vi "OutSineAmpSet.vi"(0 "SR865 in":T1, 2 "Amplitude":dbl caption="Amplitude, V", 5 "error in":errorcluster) -> (14 "SR865 out":T1, 19 "error out":errorcluster)   [LabVIEW 2018]
uses:
  SR865.ctl
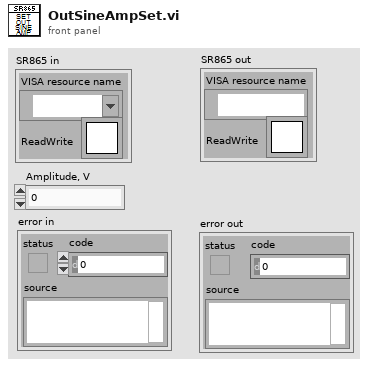
[diagram p1: front panel]
types:
  T1 = typedef "SR865.ctl" = cluster{"VISA resource name":refnum<visa-resource-name>, "ReadWrite":T2}
  T2 = typedef "Semaphore RefNum" = refnum<k1>
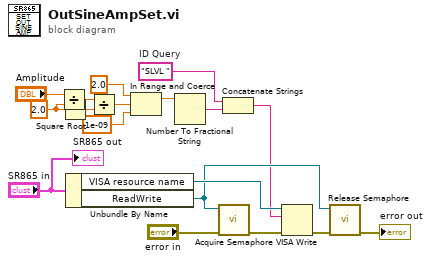
[diagram p0: block diagram]
diagram:
  w3 = 2.0 ("y")
  w9 = "SLVL "  # ID Query
  n1 = Divide(x="Amplitude", y=w3) -> (x/y=w5:dbl)
  n2 = Square Root(x=w3) -> (sqrt(x)=w4:dbl)
  n3 = Unbundle By Name("SR865 in") -> ("VISA resource name"=w17:refnum<visa-resource-name>, "ReadWrite"=w13:T2)
  n4 = Divide(x=w5, y=w4) -> (x/y=w2:dbl)
  n5 = In Range and Coerce(upper limit=2.0, x=w2, lower limit=1e-09) -> (coerced(x)=w10:dbl)  [unwired: 1 out]
  n6 = Number To Fractional String(number=w10) -> (F-format string=w8:string)  [unwired: 3 in]
  n7 = call <vilib>:"Acquire Semaphore.vi"("error in (no error)"="error in", "semaphore"=w13) -> ("error out"=w16:errorcluster)  [unwired: 3 in, 2 out]
  n8 = Concatenate Strings(w9, w8) -> (w7:string)
  n9 = VISA Write(VISA resource name=w17, write buffer=w7, error in (no error)=w16) -> (error out=w6:errorcluster)  [unwired: 2 out]
  n10 = call <vilib>:"Release Semaphore.vi"("error in (no error)"=w6, "semaphore"=w13) -> ("error out"=→"error out":errorcluster)  [unwired: 4 in, 1 out]
  "SR865 out" <- "SR865 in"
